vi "ep_Get Spectra Calibrations Points.vi"(0 "Calibration":T2={"voltage"={"full-range RMS values"=[5.0, 5.0, 5.0], "time domain"={"ranges to calibrate [%]"=[100.0], "offsets"=[0.0, 0.0, 0.0], "gains"=[[1.0], [1.0], [1.0]]}, "frequency domain"={"ranges to calibrate [%]"=[100.0], "frequencies to calibrate [Hz]"=[50.0], "phase delays [deg]"=[[[0.0]], [[0.0]], [[0.0]]], "gains"=[[[1.0]], [[1.0]], [[1.0]]]}}, "current"={"full-range RMS values"=[300.0, 300.0, 300.0, 300.0], "time domain"={"ranges to calibrate [%]"=[100.0], "offsets"=[0.0, 0.0, 0.0, 0.0], "gains"=[[1.0], [1.0], [1.0], [1.0]]}, "frequency domain"={"ranges to calibrate [%]"=[100.0], "frequencies to calibrate [Hz]"=[50.0], "phase delays [deg]"=[[[0.0]], [[0.0]], [[0.0]], [[0.0]]], "gains"=[[[1.0]], [[1.0]], [[1.0]], [[1.0]]]}}}, 7 "nominal frequency":dbl=50.0) -> (2 "voltage harmonics":dbl[][](array[numeric]), 3 "current harmonics":dbl[][](array[numeric]), 4 "voltages#":i32, 6 "voltages RMS":dbl[](array[numeric]), 8 "currents RMS":dbl[](array[numeric]), 10 "harmonics":T1(array[cluster]), 14 "spectra indexees":i32[](array[numeric]), 15 "harmonics states":bool[](array[boolean]))   [LabVIEW 2012]
uses:
  <vilib>/addons/Electrical Power/Example Support/PQ/Calibration/ep_Calibration.ctl
panel:
  out "RMS":dbl[](array[numeric])
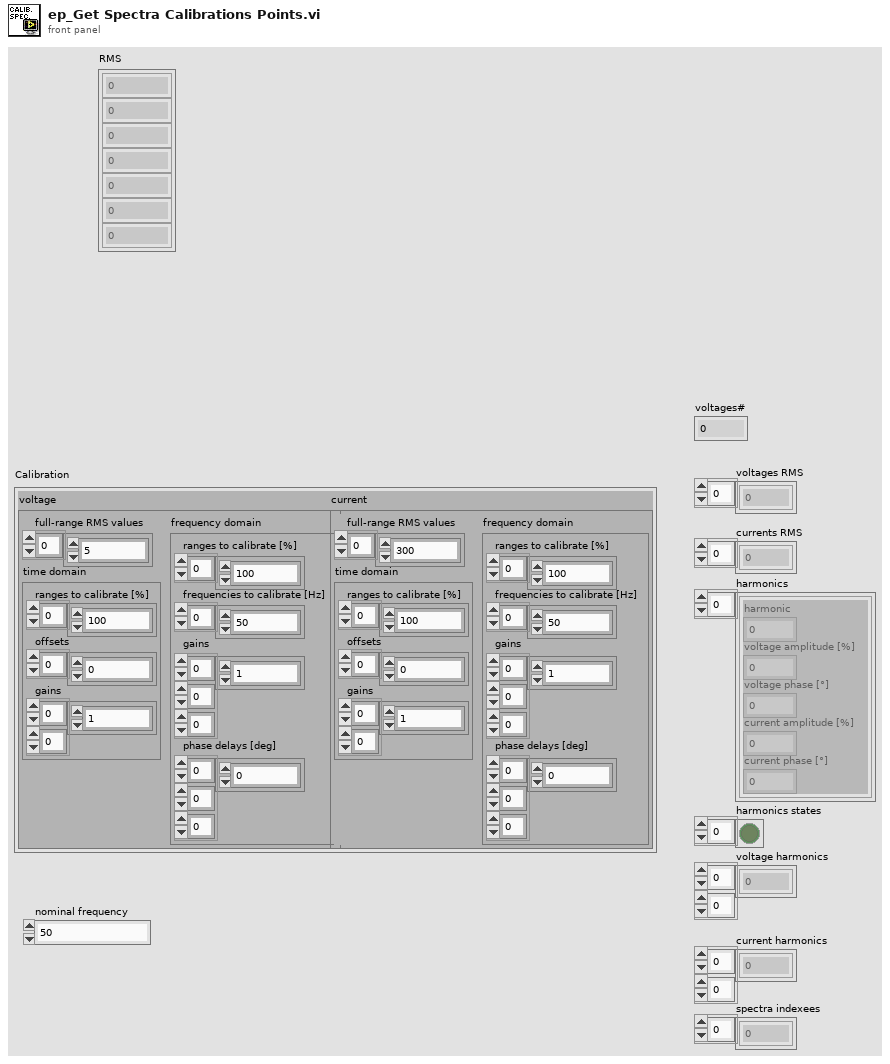
[diagram p1: front panel]
types:
  T1 = cluster{"harmonic":u32, "voltage amplitude [%]":dbl, "voltage phase [°]":dbl, "current amplitude [%]":dbl, "current phase [°]":dbl}[]
  T2 = typedef "ep_Calibration.ctl" = cluster{"voltage":cluster{"full-range RMS values":dbl[], "time domain":cluster{"ranges to calibrate [%]":dbl[], "offsets":dbl[], "gains":dbl[][]}, "frequency domain":cluster{"ranges to calibrate [%]":dbl[], "frequencies to calibrate [Hz]":dbl[], "phase delays [deg]":dbl[][][], "gains":dbl[][][]}}, "current":cluster{"full-range RMS values":dbl[], "time domain":cluster{"ranges to calibrate [%]":dbl[], "offsets":dbl[], "gains":dbl[][]}, "frequency domain":cluster{"ranges to calibrate [%]":dbl[], "frequencies to calibrate [Hz]":dbl[], "phase delays [deg]":dbl[][][], "gains":dbl[][][]}}}
  T3 = cluster{"harmonic":u32, "voltage amplitude [%]":dbl, "voltage phase [°]":dbl, "current amplitude [%]":dbl, "current phase [°]":dbl}
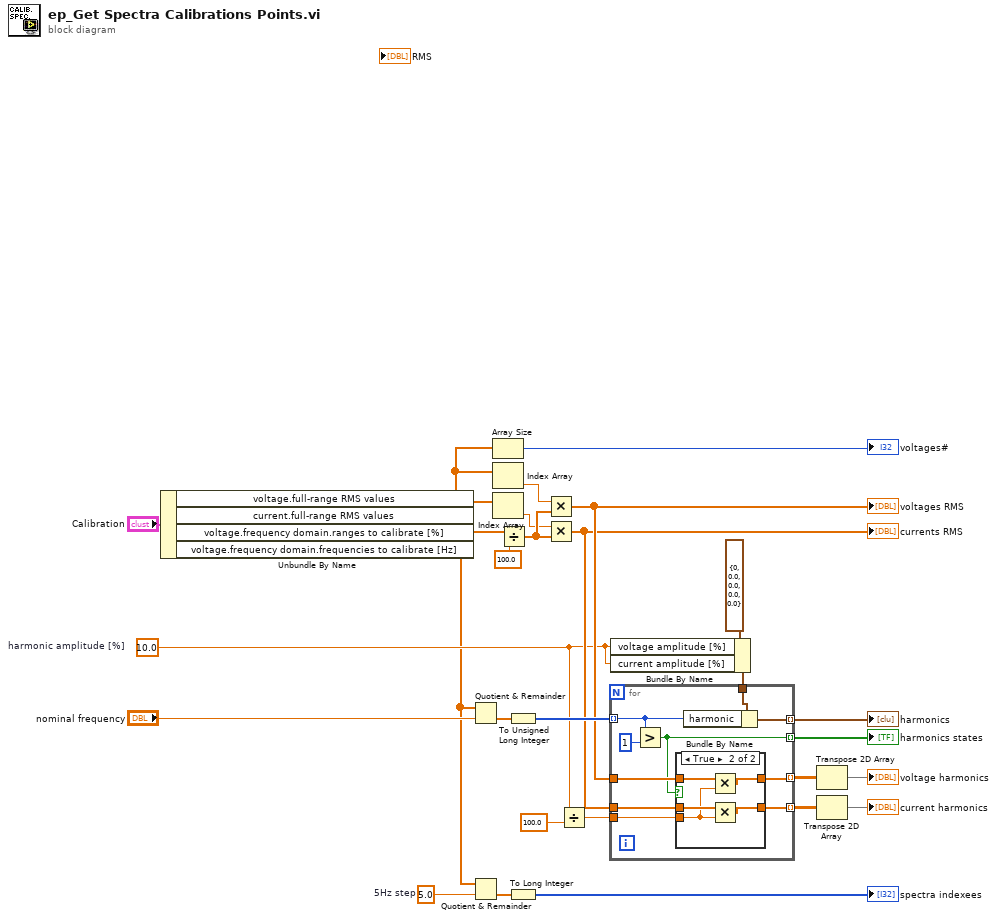
[diagram p0: block diagram]
diagram:
  w4 = 5.0  # 5Hz step
  w11 = 10.0  # harmonic amplitude [%]
  n1 = Unbundle By Name("Calibration") -> ("voltage.full-range RMS values"=w24:dbl[], "current.full-range RMS values"=w22:dbl[], "voltage.frequency domain.ranges to calibrate [%]"=w26:dbl[], "voltage.frequency domain.frequencies to calibrate [Hz]"=w2:dbl[])
  n2 = Quotient & Remainder(x=w2, y="nominal frequency") -> (floor(x/y)=w5:dbl[])  [unwired: 1 out]
  n3 = Quotient & Remainder(x=w2, y=w4) -> (floor(x/y)=w3:dbl[])  [unwired: 1 out]
  n4 = Array Size(array=w24) -> (size(s)=→"voltages#":i32)
  n5 = Index Array(array=w24) -> (element=w23:dbl)  [unwired: 1 in]
  n6 = Index Array(array=w22) -> (element=w21:dbl)  [unwired: 1 in]
  n7 = Divide(x=w26, y=100.0 ("element")) -> (x/y=w28:dbl[])
  n8 = To Unsigned Long Integer(number=w5) -> (unsigned 32bit integer=w19:u32[])
  n9 = To Long Integer(number=w3) -> (32bit integer=→"spectra indexees":i32[])
  n10 = Multiply(x=w23, y=w28) -> (x*y=w16:dbl[])
  "voltages RMS" <- w16
  n11 = Multiply(x=w21, y=w28) -> (x*y=w15:dbl[])
  "currents RMS" <- w15
  n12 = Divide(x=w11, y=100.0) -> (x/y=w13:dbl)
  n13 = Bundle By Name(cluster=T3 {"harmonic"=0, "voltage amplitude [%]"=0.0, "voltage phase [°]"=0.0, "current amplitude [%]"=0.0, "current phase [°]"=0.0} ("voltage harmonic"), "voltage amplitude [%]"=w11, "current amplitude [%]"=w11) -> (w10:T3)
  n14 = for {
    tunnel: w19 -> [w38] mode=indexing
    tunnel: [w39] -> w18 mode=indexing
    tunnel: [w30] -> w17 mode=indexing
    tunnel: w16 -> [w36]
    tunnel: w15 -> [w35]
    tunnel: w13 -> [w34]
    tunnel: w10 -> [w33]
    tunnel: [w32] -> w9 mode=indexing
    tunnel: [w31] -> w8 mode=indexing
    n15 = Greater?(x=w38, y=u32 1 ("x")) -> (0:w30:bool)
    n16 = case shown="True" w30 {
      tunnel: w36 -> [w41 w46]
      tunnel: w35 -> [w40 w45]
      tunnel: w34 -> [_ w44]
      tunnel: [w41 w43] -> w32
      tunnel: [w40 w42] -> w31
      frame False {
      }
      frame True {
        n17 = Multiply(x=w46, y=w44) -> (x*y=w43:dbl[])
        n18 = Multiply(x=w45, y=w44) -> (x*y=w42:dbl[])
      }
    }
    n19 = Bundle By Name(cluster=w33, "harmonic"=w38) -> (w39:T3)
  }
  "harmonics" <- w18
  "harmonics states" <- w17
  n20 = Transpose 2D Array(2D array=w9) -> (transposed array=→"voltage harmonics":dbl[][])
  n21 = Transpose 2D Array(2D array=w8) -> (transposed array=→"current harmonics":dbl[][])
